vi "Variable globale 1.vi"() -> ()   [LabVIEW 2010]
panel:
  in  "stopglob":bool
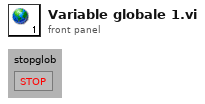
[diagram p1: front panel]
diagram:
